vi "modify channel test.vi"() -> ()   [LabVIEW 2013, in "UI reference module tests.lvlib"]
uses:
  UI reference module tests.lvlib
  <vilib>/NI/Tag Bus Module Framework/channel/TBM channel.lvclass/TBM channel.ctl
  <vilib>/NI/Tag Bus Module Framework/channel/channel classification.ctl
  module/configuration/UI Reference configuration.lvclass
  <vilib>/NI/Tag Bus/tag/tag descriptor.lvclass/tag descriptor.ctl
  <vilib>/NI/Tag Bus Module Framework/channel/Read channel classification.vi
  <vilib>/NI/Tag Bus Module Framework/channel/Write channel classification.vi
  <vilib>/NI/Tag Bus/tag/read tag name.vi
  <vilib>/NI/Tag Bus Module Framework/channel/TBM channel.lvclass
panel:
  out "mod success":bool
  out "no err":errorcluster
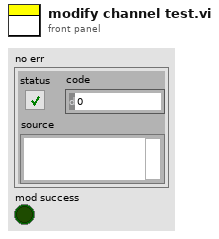
[diagram p1: front panel]
types:
  T1 = typedef "TBM channel.lvclass/channel classification.ctl" = enum16{"input data", "output data", "processing parameter", "processing result"}
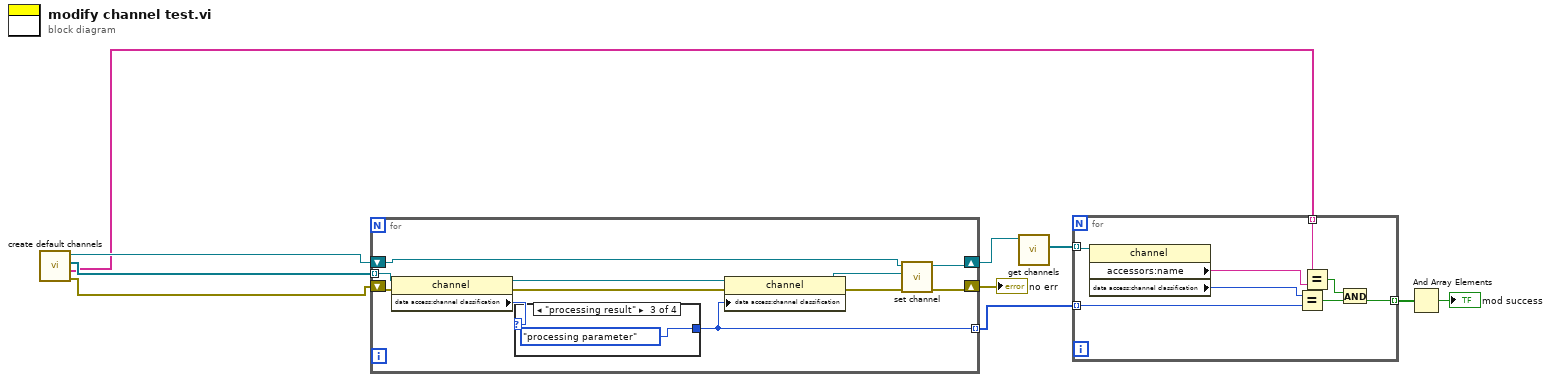
[diagram p0: block diagram]
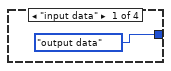
[diagram p2: hidden frame]
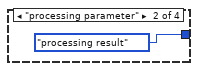
[diagram p3: hidden frame]
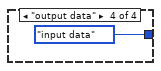
[diagram p4: hidden frame]
diagram:
  n1 = call "create default channels.vi"() -> ("error out"=w2:errorcluster, "names"=w1:string[], "channels"=w3:refnum<class "TBM channel.lvclass">[], "module"=w4:refnum<class "UI Reference configuration.lvclass">)  [unwired: 7 in, 1 out]
  n2 = for {
    shift-right: [w20] -> w10
    shift-left: w4 -> [w21]
    shift-right: [w19] -> w9
    shift-left: w2 -> [w18]
    tunnel: w3 -> [w16] mode=indexing
    tunnel: [w11] -> w5 mode=indexing
    n3 = property class="channel"(reference=w16, error in=w18) -> (reference out=w14:refnum<class "TBM channel.lvclass">, error out=w17:errorcluster, "data access:channel classification"=w12:T1)
    n4 = case shown="\"processing result\"" w12 {
      tunnel: [channel_classification."output data" ("channel classification") channel_classification."processing result" ("channel classification") channel_classification."processing parameter" ("channel classification") channel_classification."input data" ("channel classification")] -> w11
      frame "input data" {
      }
      frame "processing parameter" {
      }
      frame "processing result" {
      }
      frame "output data" {
      }
    }
    n5 = property class="channel"(reference=w14, error in=w17, "data access:channel classification"=w11) -> (reference out=w13:refnum<class "TBM channel.lvclass">, error out=w15:errorcluster)
    n6 = call "set channel.vi"("error in"=w15, "channel"=w13, "UI Reference configuration in"=w21) -> ("error out"=w19:errorcluster, "UI Reference configuration out"=w20:refnum<class "UI Reference configuration.lvclass">)  [unwired: 7 in]
  }
  "no err" <- w9
  n7 = call-dynamic "get channels.vi"("UI Reference configuration in"=w10) -> ("channels"=w8:refnum<class "TBM channel.lvclass">[])  [unwired: 9 in, 1 out]
  n8 = for {
    tunnel: w8 -> [w32] mode=indexing
    tunnel: [w31] -> w7 mode=indexing
    tunnel: w5 -> [w30] mode=indexing
    tunnel: w1 -> [w27] mode=indexing
    n9 = property class="channel"(reference=w32) -> ("accessors:name"=w28:string, "data access:channel classification"=w29:T1)  [unwired: 1 in, 2 out]
    n10 = Equal?(x=w29, y=w30) -> (x = y?=w33:bool)
    n11 = Equal?(x=w27, y=w28) -> (x = y?=w26:bool)
    n12 = And(x=w26, y=w33) -> (x .and. y?=w31:bool)
  }
  n13 = And Array Elements(Boolean array=w7) -> (logical AND=→"mod success":bool)
